vi "MTIF_Read_Smart.vi"(8 "error in":errorcluster, 9 "Input Parameters":T3={"Drop Bits"=0, "Output Files?"=TRUE, "STD Threshold Ratio for Start"=1.2, "STD Threshold Ratio for Stop"=1.1, "Output Image Type"=0, "Timeout for Queue(ms)"=1000, "Output Queue?"=FALSE, "Output File Format"=enum."TIFF", "Initial STD Threshold"=65535.0, "Number of Buffered Frames"=150, "Centroid Distence Threshold"=1.0} {"Output Image Type" items=["Grayscale (U8)", "Grayscale (I16)", "Grayscale (SGL)", "Complex (CSG)", "RGB (U32)", "HSL (U32)", "RGB (U64)", "Grayscale (U16)"]}, 10 "File Name (.mtif)":string="zebrafish_7", 11 "Folder Path":path=path "X:/Zebrafish_VR_Data") -> (0 "error out":errorcluster, 2 "Manual ROI":T1={"Global Rectangle"=[143, 107, 365, 263], "Contours"=[{"Contour Type"=0, "ROI Type"=4, "Points"=[143, 107, 365, 263]}]}, 3 "U16 Array Queue Out":refnum<queue>)   [LabVIEW 2014]
uses:
  <vilib>/vision/NI_Vision_Development_Module.lvlib
panel:
  out "Buffer Full?":bool=TRUE
  out "Standard Variation":sgl=42.84885
  out "Centroid":cluster{"X Centroid":sgl, "Y Centroid":sgl}={"X Centroid"=249.5989, "Y Centroid"=187.47522} {"Y Centroid" format="%.2f"; "X Centroid" format="%.2f"}
  in  "Stop":bool
  out "Frame No.":i32=996
  out "Sequence No.":u16
  out "Progress":dbl=1.0000000032682703 format="%#.3f"
  out "Data Valid?":bool=TRUE
  out "Raw Image":T4(plugin-control)
  out "Frame Rate":dbl=550.0
  out "File ROI":T5={"Left"=0, "Top"=0, "Right"=639, "Bottom"=479, "Rotation"=0.0} {"Rotation" format="%.2f"; "Left" scale=0.0..1024.0; "Right" scale=0.0..1024.0}
  # "Max 2GB\nfor one AVI file!"
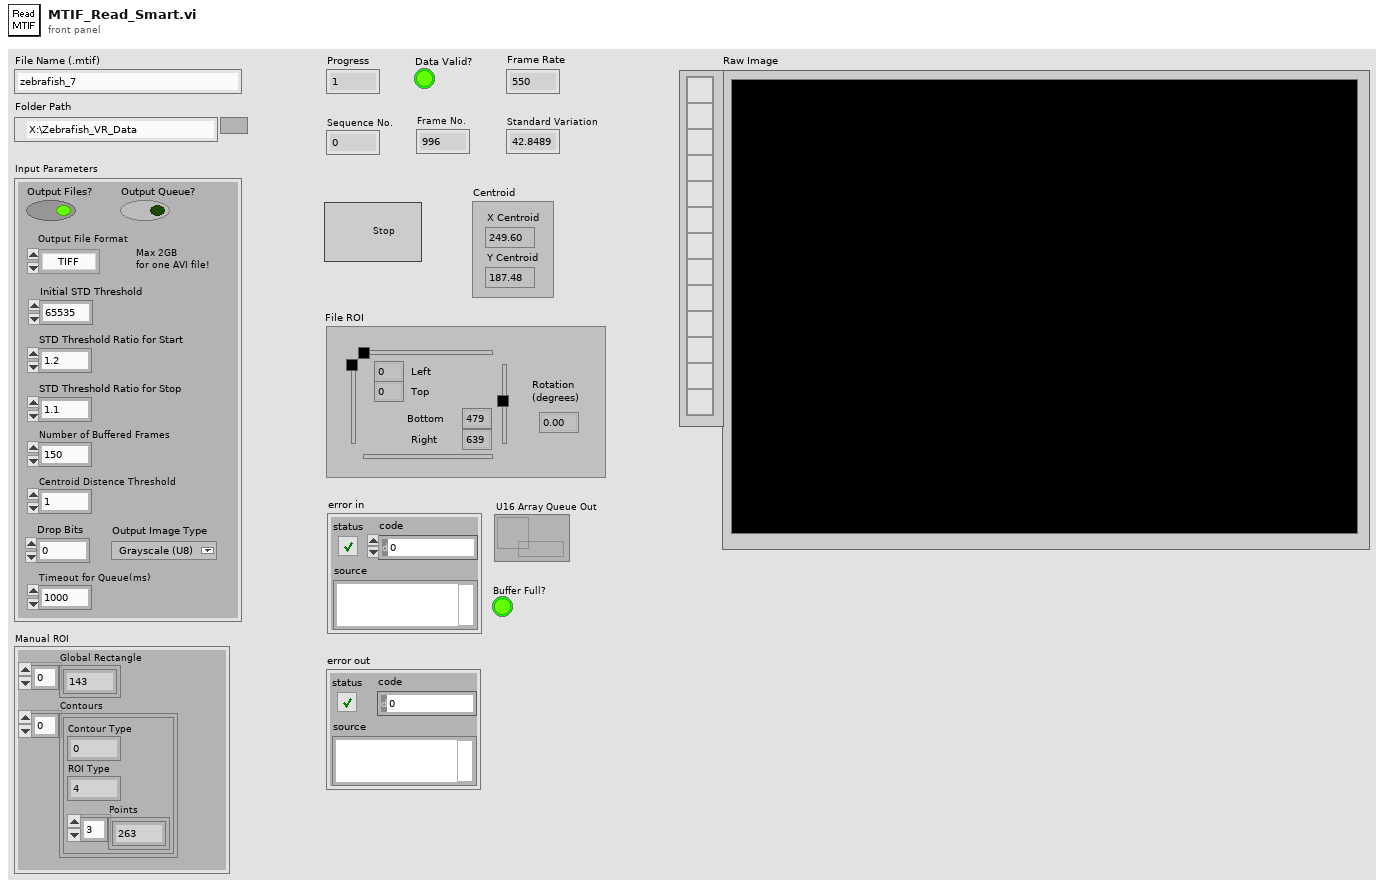
[diagram p1: front panel]
types:
  T1 = cluster{"Global Rectangle":i32[], "Contours":cluster{"Contour Type":u32, "ROI Type":u32, "Points":i32[]}[]}
  T2 = typedef "Image Type" = u32
  T3 = cluster{"Drop Bits":i8, "Output Files?":bool, "STD Threshold Ratio for Start":dbl, "STD Threshold Ratio for Stop":dbl, "Output Image Type":T2, "Timeout for Queue(ms)":u32, "Output Queue?":bool, "Output File Format":enum16{"TIFF", "AVI"}, "Initial STD Threshold":sgl, "Number of Buffered Frames":i32, "Centroid Distence Threshold":sgl}
  T4 = typedef "IMAQ Image.ctl" = refnum<image>
  T5 = typedef "IMAQ Rectangle" = cluster{"Left":i32, "Top":i32, "Right":i32, "Bottom":i32, "Rotation":dbl}
  T6 = cluster{"ImgDataArray":u16[][], "Centroid":cluster{"X Centroid":sgl, "Y Centroid":sgl}, "Frame No.":i32, "Standard Variation":sgl}
  T7 = enum16{"big-endian, network order", "native, host order", "little-endian"}
  T8 = enum16{"open", "replace", "create", "open or create", "replace or create", "replace or create with confirmation"}
  T9 = cluster{"[0]":i32, "[1]":i32, "[2]":i32, "[3]":i32}
  T10 = cluster{"Global Rectangle":i32[], "Contours":cluster{"Contour Type":u32, "Type":u32, "Coordinates":i32[]}[]}
  T11 = cluster{"Mean Value":sgl, "Standard Variation":sgl, "Minimal Value":sgl, "Maximal Value":sgl, "Area (calibrated)":sgl, "Area (pixels)":u32, "%":sgl, "Calibration Valid":bool}
  T12 = typedef "IMAQ AVI2 Refnum.ctl" = refnum<k20>
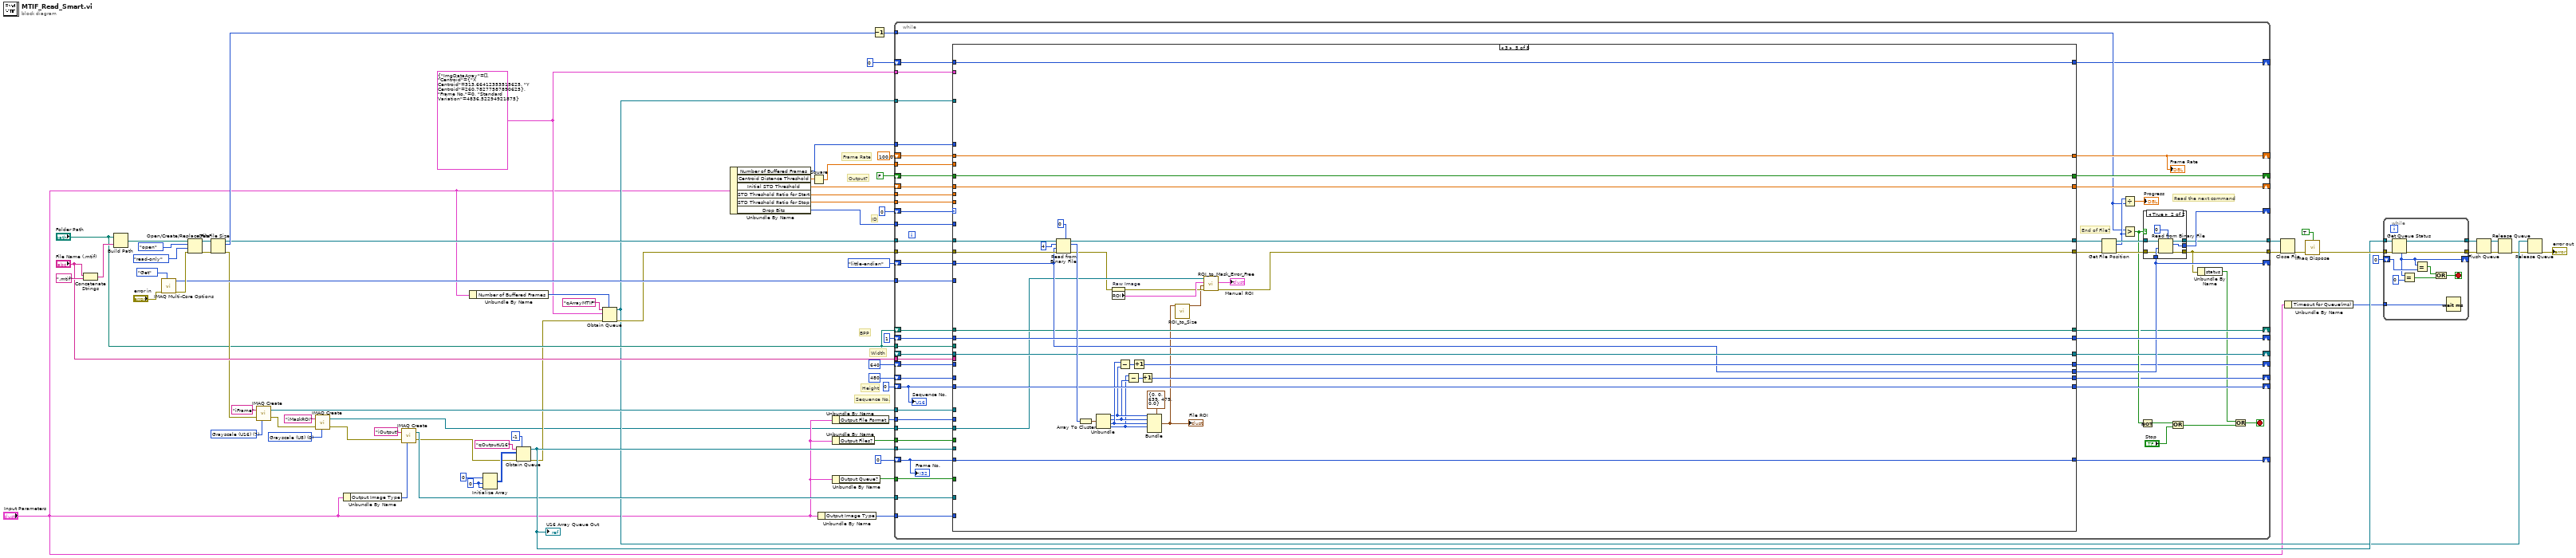
[diagram p0: block diagram]
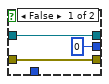
[diagram p2: hidden frame]
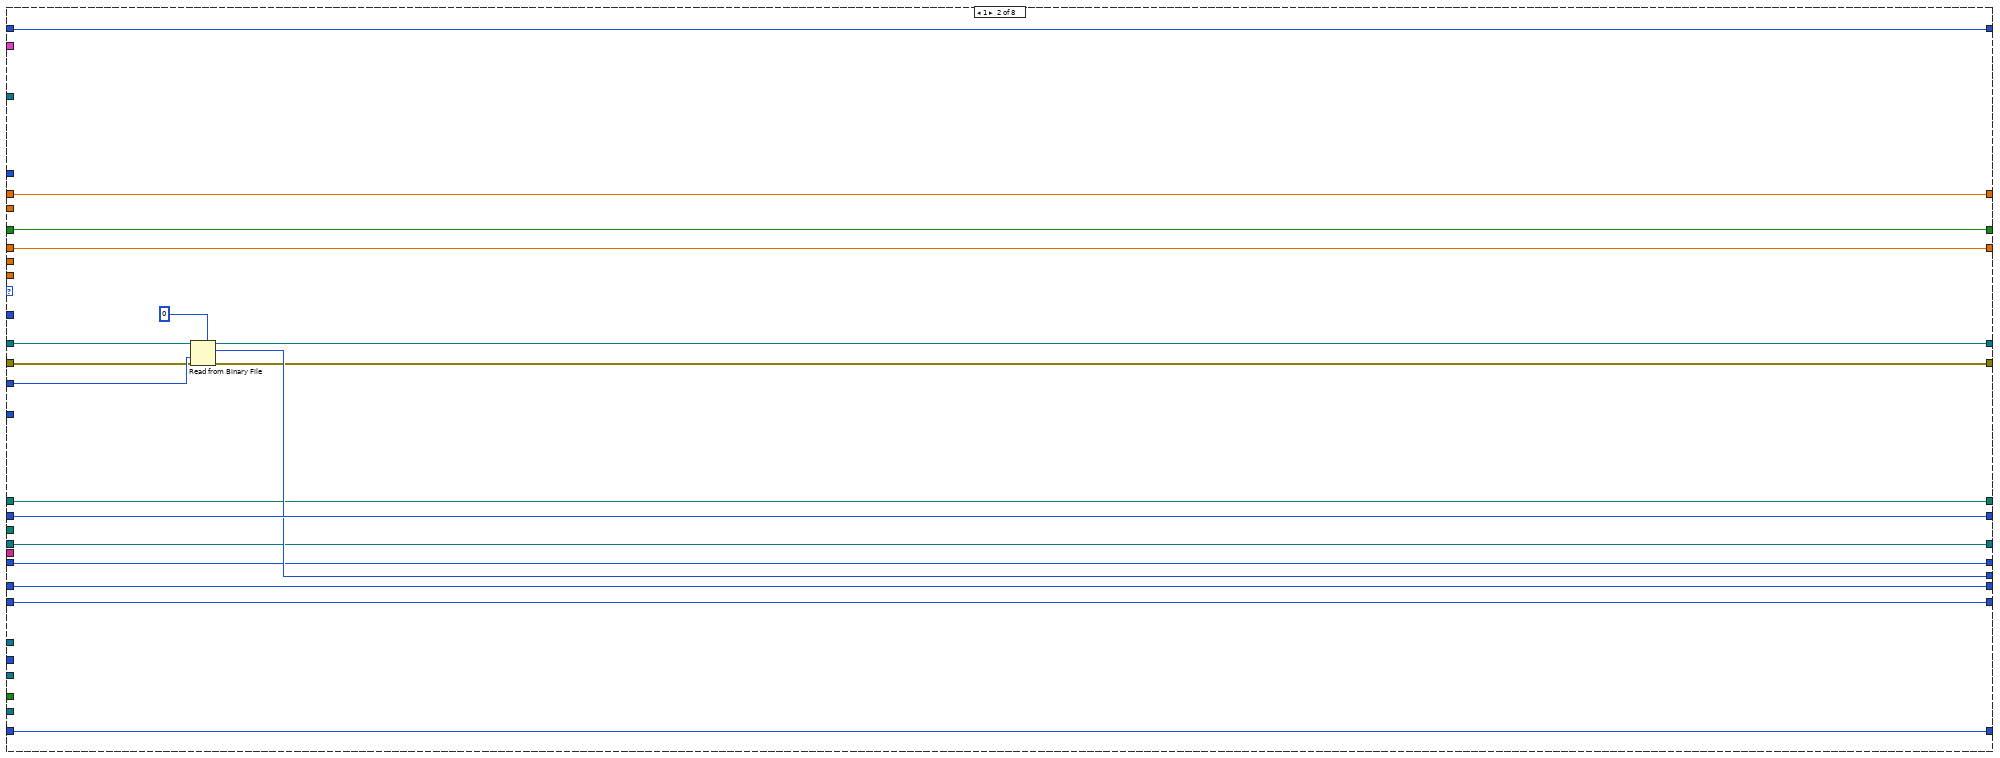
[diagram p4: hidden frame]
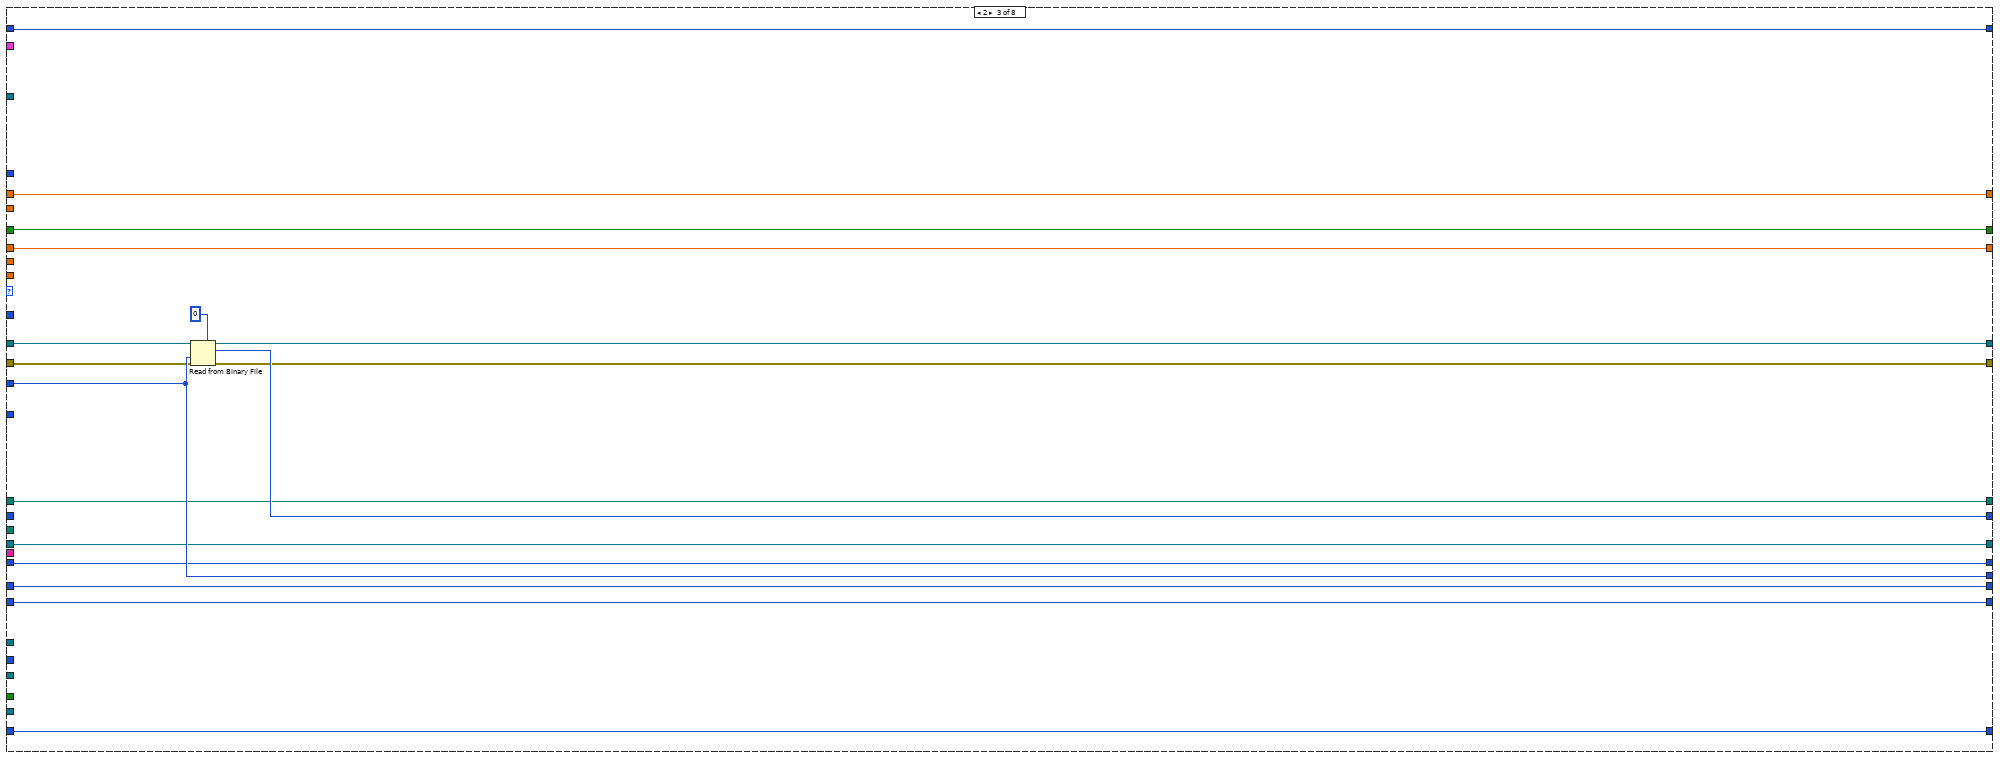
[diagram p5: hidden frame]
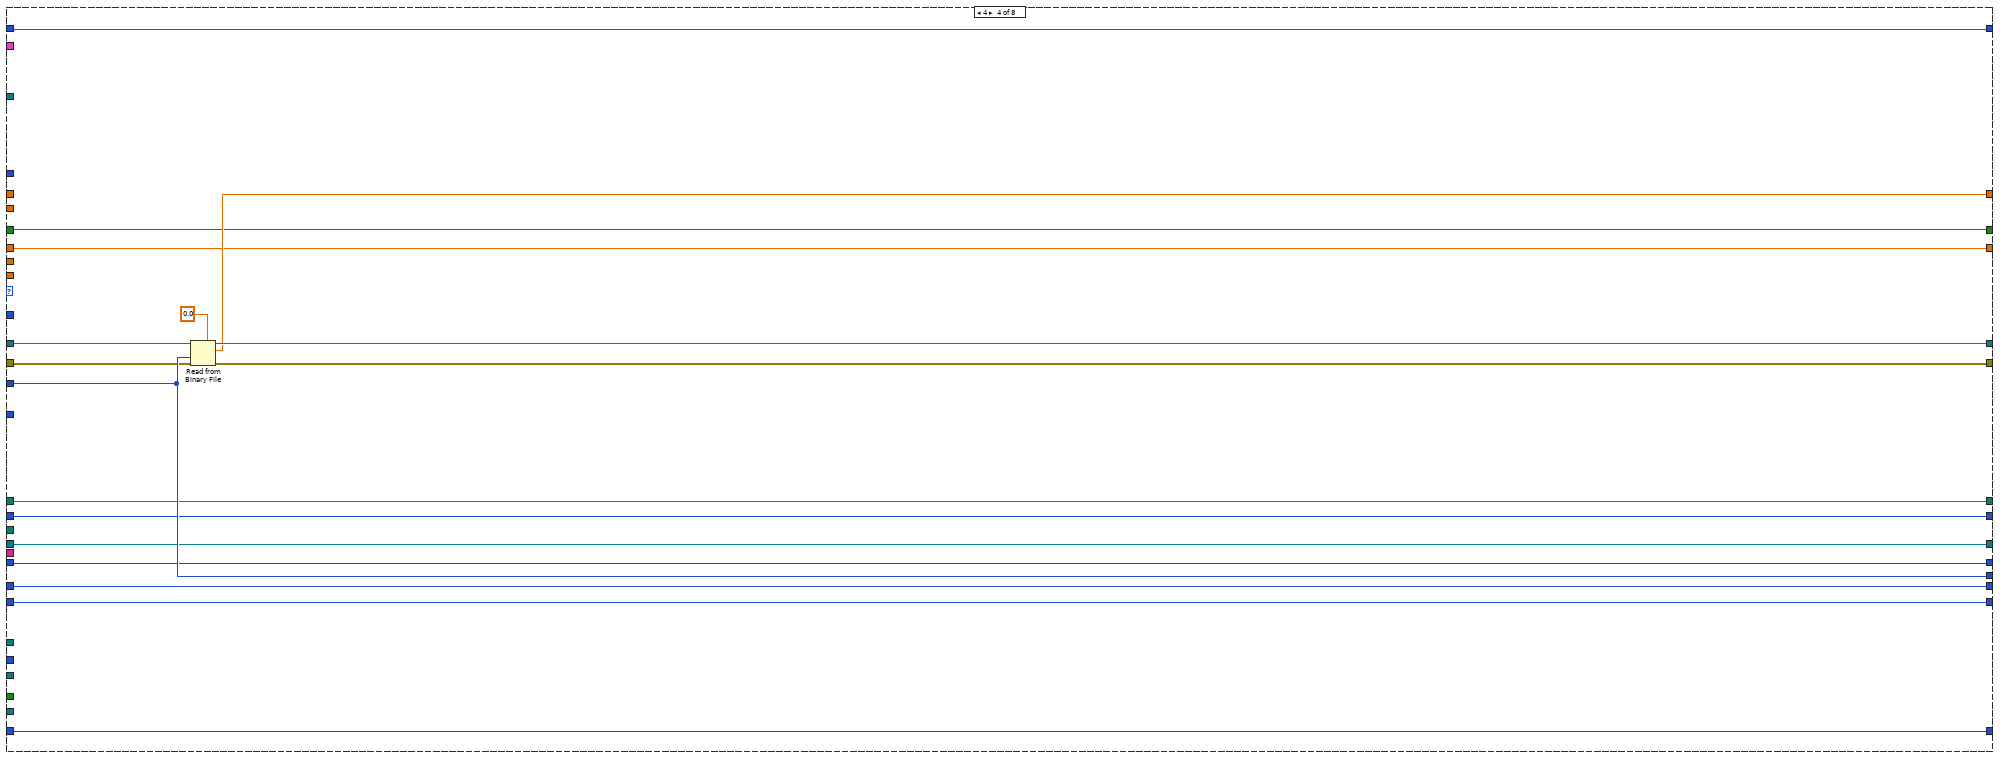
[diagram p6: hidden frame]
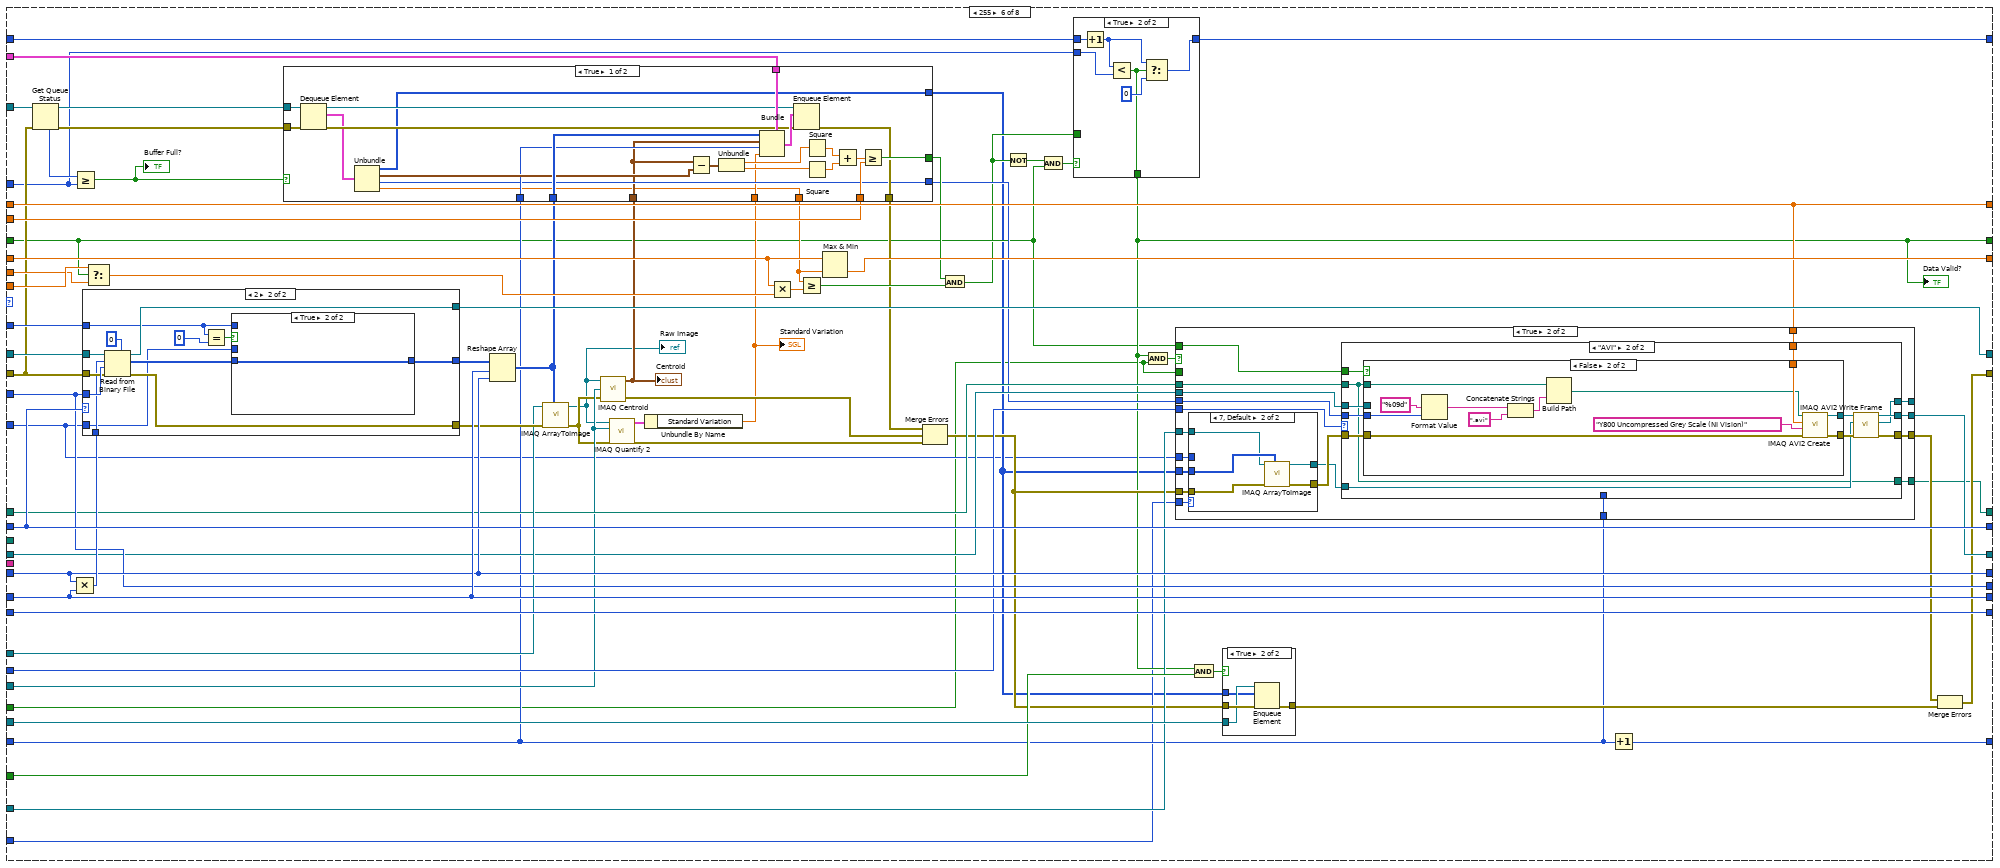
[diagram p7: hidden frame]
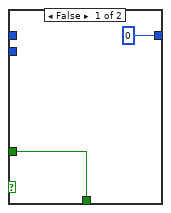
[diagram p8: hidden frame]
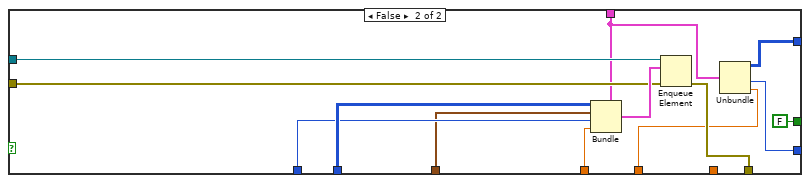
[diagram p9: hidden frame]
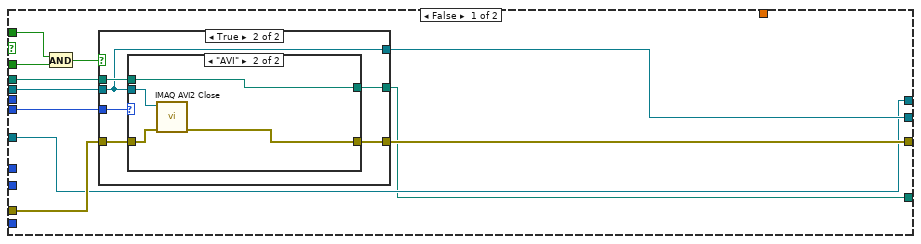
[diagram p11: hidden frame]
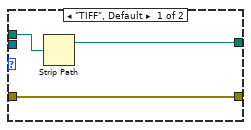
[diagram p13: hidden frame]
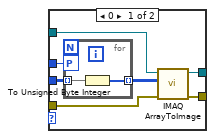
[diagram p14: hidden frame]
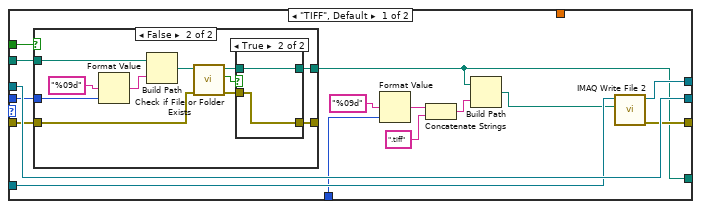
[diagram p15: hidden frame]
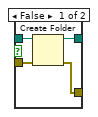
[diagram p17: hidden frame]
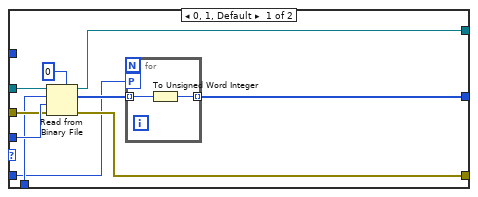
[diagram p19: hidden frame]
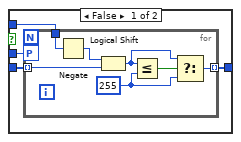
[diagram p20: hidden frame]
diagram:
  w13 = T6 {"ImgDataArray"=[], "Centroid"={"X Centroid"=313.66412, "Y Centroid"=260.78278}, "Frame No."=0, "Standard Variation"=4836.523}
  w24 = T2 0 items=["Grayscale (U8)", "Grayscale (I16)", "Grayscale (SGL)", "Complex (CSG)", "RGB (U32)", "HSL (U32)", "RGB (U64)", "Grayscale (U16)"] ("Image Type")
  w25 = T2 7 items=["Grayscale (U8)", "Grayscale (I16)", "Grayscale (SGL)", "Complex (CSG)", "RGB (U32)", "HSL (U32)", "RGB (U64)", "Grayscale (U16)"] ("Image Type")
  w20 = 0 ("dimension size")
  # "Output?"
  # "Sequence No."
  # "Height"
  # "Width"
  # "BPP"
  # "ID"
  # "Frame Rate"
  n1 = Concatenate Strings("File Name (.mtif)", ".mtif" ("string")) -> (w73:string)
  n2 = Build Path(base path="Folder Path", name or relative path=w73) -> (appended path=w69:path)
  n3 = call "IMAQ Multi-Core Options"("Get/Set Number of Cores (Get)"=enum32{"Get", "Set", "Set Max Available"}."Get", "error in (no error)"="error in") -> ("error out"=w59:errorcluster, "Cores Utilized"=w58:u32)  [unwired: 8 in]
  n4 = Open/Create/Replace File(file path (use dialog)=w69, error in=w59, operation (0:open)=T8."open", access (0:read/write)=enum16{"read/write", "read-only", "write-only"}."read-only") -> (refnum out=w64:refnum<file>, error out=w65:errorcluster)  [unwired: 2 in, 1 out]
  n5 = Get File Size(file=w64, error in=w65) -> (refnum out=w55:refnum<file>, size (in bytes)=w63:i64, 0:w53:errorcluster)
  n6 = call "IMAQ Create"("Image Name"="iFrame", "Image Type"=w25, "error in (no error)"=w53) -> ("New Image"=w52:T4, "error out"=w51:errorcluster)  [unwired: 2 in]
  n7 = call "IMAQ Create"("Image Name"="iMaskROI", "Image Type"=w24, "error in (no error)"=w51) -> ("New Image"=w2:T4, "error out"=w3:errorcluster)  [unwired: 2 in]
  n8 = Unbundle By Name("Input Parameters") -> ("Output Image Type"=w22:T2)
  n9 = call "IMAQ Create"("Image Name"="iOutput", "Image Type"=w22, "error in (no error)"=w3) -> ("New Image"=w21:T4, "error out"=w1:errorcluster)  [unwired: 2 in]
  n10 = Unbundle By Name("Input Parameters") -> ("Number of Buffered Frames"=w15:i32)
  n11 = Initialize Array(u16 0 ("element"), w20, w20) -> (w44:u16[][])
  n12 = Obtain Queue(max queue size (-1, unlimited)=-1, name (unnamed)="qOutputU16", element data type=w44, error in (no error)=w1) -> (queue out=w35:refnum<queue>, error out=w16:errorcluster)  [unwired: 1 in, 1 out]
  "U16 Array Queue Out" <- w35
  n13 = Obtain Queue(max queue size (-1, unlimited)=w15, name (unnamed)="qArrayMTIF", element data type=w13, error in (no error)=w16) -> (queue out=w9:refnum<queue>, error out=w14:errorcluster)  [unwired: 1 in, 1 out]
  n14 = Unbundle By Name("Input Parameters") -> ("Number of Buffered Frames"=w18:i32, "Centroid Distence Threshold"=w11:sgl, "Initial STD Threshold"=w19:sgl, "STD Threshold Ratio for Start"=w32:dbl, "STD Threshold Ratio for Stop"=w30:dbl, "Drop Bits"=w29:i8)
  n15 = Square(x=w11) -> (x^2=w10:sgl)
  n16 = Unbundle By Name("Input Parameters") -> ("Output Image Type"=w4:T2)
  n17 = Unbundle By Name("Input Parameters") -> ("Output File Format"=w28:enum16{"TIFF", "AVI"})
  n18 = Unbundle By Name("Input Parameters") -> ("Output Files?"=w34:bool)
  n19 = Unbundle By Name("Input Parameters") -> ("Output Queue?"=w33:bool)
  n20 = Decrement(x=w63) -> (x-1=w62:i64)
  n21 = while {
    shift-right: [w130] -> _
    shift-left: u8 0 -> [w137]
    shift-right: [w135] -> _
    shift-left: u8 1 -> [w136]
    tunnel: w55 -> [w134]
    shift-right: [w132] -> _
    shift-left: T7."little-endian" ("Byte Order") -> [w133]
    tunnel: w14 -> [w131]
    tunnel: [w80] -> w47
    shift-right: [w128] -> _
    shift-left: 100.0 -> [w129]
    shift-right: [w122] -> _
    shift-left: u16 0 -> [w127]
    shift-right: [w124] -> _
    shift-left: _ -> [w123]
    tunnel: w62 -> [w100]
    shift-right: [w116] -> _
    shift-left: 640 -> [w114]
    shift-right: [w115] -> _
    shift-left: 480 -> [w113]
    tunnel: w29 -> [w112]
    tunnel: w58 -> [w111]
    tunnel: w52 -> [w110]
    tunnel: w34 -> [w102]
    tunnel: w2 -> [w109]
    shift-right: [w106] -> _
    shift-left: w19 -> [w107]
    shift-right: [w104] -> _
    shift-left: FALSE -> [w108]
    tunnel: w30 -> [w105]
    tunnel: w32 -> [w103]
    tunnel: [w98] -> w46
    tunnel: "Folder Path" -> [w126]
    tunnel: w35 -> [w97]
    tunnel: w33 -> [w96]
    tunnel: w28 -> [w95]
    tunnel: "File Name (.mtif)" -> [w125]
    shift-right: [w93] -> _
    shift-left: "Folder Path" -> [w94]
    tunnel: w21 -> [w90]
    tunnel: w18 -> [w89]
    tunnel: w10 -> [w88]
    tunnel: w9 -> [w87]
    tunnel: w13 -> [w86]
    shift-right: [w84] -> _
    shift-left: 0 -> [w85]
    shift-right: [w82] -> _
    shift-left: 0 -> [w83]
    tunnel: w4 -> [w81]
    stop <- w77 stop-if-true
    # "Read the next command"
    # "End of File?"
    n22 = case shown="3" w137 {
      tunnel: w133 -> [w161 w178 w195 w212 w224 w305 w535 w597]
      tunnel: [w161 w174 w195 w212 w224 w305 w535 w597] -> w132
      tunnel: w136 -> [w160 w177 _ w206 w238 w314 w553 w592]
      tunnel: [w160 w177 w192 w206 w238 w314 w553 w592] -> w135
      tunnel: w134 -> [w159 w176 w193 w210 w245 w316 w543 w595]
      tunnel: w131 -> [w158 w175 w194 w211 w246 w272 w526 w586]
      tunnel: [w158 w173 w191 w209 w221 w290 w547 w601] -> w120
      tunnel: [w159 w172 w190 w208 w244 w304 w542 w594] -> w121
      tunnel: [w157 w171 w189 w207 w239 w293 w548 w577] -> w128
      tunnel: w129 -> [w157 w171 w189 _ w239 w293 w548 w577]
      tunnel: w127 -> [w155 w169 w187 w204 w236 w315 w532 w590]
      tunnel: w126 -> [_ _ _ _ _ _ w551 _]
      tunnel: w125 -> [_ _ _ _ _ _ w550 _]
      tunnel: [w156 w170 w188 w205 w237 w299 w531 w578] -> w124
      tunnel: w123 -> [w156 w170 w188 w205 w237 w300 w531 w578]
      tunnel: [w155 w169 w187 w204 w236 w315 w532 w589] -> w122
      tunnel: [w154 w168 w186 w203 w229 w309 w545 w599] -> w116
      tunnel: [w153 w167 w185 w202 w228 w310 w546 w600] -> w115
      tunnel: w114 -> [w154 w168 w186 w203 _ w309 w545 w599]
      tunnel: w113 -> [w153 w167 w185 w202 _ w310 w546 w600]
      tunnel: w112 -> [_ _ _ _ _ w313 _ _]
      tunnel: w111 -> [_ _ _ _ _ w249 _ w569]
      tunnel: w110 -> [_ _ _ _ _ w307 _ _]
      tunnel: w109 -> [_ _ _ _ w220 w283 _ _]
      tunnel: w108 -> [w152 w166 w184 w201 w227 w253 _ w582]
      tunnel: w107 -> [w151 w165 w183 w200 w226 w296 w528 w593]
      tunnel: [w151 w165 w183 w200 w226 w303 w528 w593] -> w106
      tunnel: w105 -> [_ _ _ _ _ w302 _ _]
      tunnel: [w152 w166 w184 w201 w227 w254 FALSE FALSE] -> w104
      tunnel: w103 -> [_ _ _ _ _ w301 _ _]
      tunnel: w102 -> [_ _ _ _ _ w248 w534 w576]
      tunnel: w85 -> [w150 w164 w182 w199 w225 w265 _ w591]
      tunnel: [w150 w164 w182 w199 w225 w294 0 w591] -> w84
      tunnel: w97 -> [_ _ _ _ _ w292 _ w574]
      tunnel: w96 -> [_ _ _ _ _ w287 _ w575]
      tunnel: w95 -> [_ _ _ _ _ w286 _ w579]
      tunnel: w94 -> [w149 w163 w181 w198 w223 w285 _ w570]
      tunnel: [w149 w163 w181 w198 w223 w284 w529 w570] -> w93
      tunnel: w90 -> [_ _ _ _ _ w267 _ w573]
      tunnel: w89 -> [_ _ _ _ _ w255 _ _]
      tunnel: w88 -> [_ _ _ _ _ w277 _ _]
      tunnel: w87 -> [_ _ _ _ _ w274 w527 w587]
      tunnel: w86 -> [_ _ _ _ _ w263 _ _]
      tunnel: w83 -> [w148 w162 w180 w197 w222 w257 _ _]
      tunnel: [w148 w162 w180 w197 w222 w256 0 ("f") 0 ("f")] -> w82
      tunnel: w81 -> [_ _ _ _ _ w251 _ w580]
      frame 0, Default {
      }
      frame 1 {
        n23 = Read from Binary File(5:u8 0, 8:w175, 9:w178, 11:w176) -> (0:w173:errorcluster, 2:w174:u8, 3:w172:refnum<file>)  [unwired: 2 in, 1 out]
      }
      frame 2 {
        n24 = Read from Binary File(5:u8 0, 8:w194, 9:w195, 11:w193) -> (0:w191:errorcluster, 2:w192:u8, 3:w190:refnum<file>)  [unwired: 2 in, 1 out]
      }
      frame 4 {
        n25 = Read from Binary File(5:0.0, 8:w211, 9:w212, 11:w210) -> (0:w209:errorcluster, 2:w207:dbl, 3:w208:refnum<file>)  [unwired: 2 in, 1 out]
      }
      frame 3 {
        n26 = Read from Binary File(5:0, 8:w246, 9:w224, 10:4 ("count (1)"), 11:w245) -> (0:w217:errorcluster, 2:w242:i32[], 3:w244:refnum<file>)  [unwired: 1 in, 1 out]
        n27 = Array To Cluster(array=w242) -> (cluster=w241:T9)
        n28 = Unbundle(w241) -> ("[0]"=w232:i32, "[1]"=w231:i32, "[2]"=w233:i32, "[3]"=w230:i32)
        n29 = property on="Raw Image" class="ImageControl"(error in=w217) -> (error out=w216:errorcluster, "ROI"=w219:T1)  [unwired: 1 in, 1 out]
        n30 = Subtract(x=w233, y=w232) -> (x-y=w234:i32)
        n31 = Subtract(x=w230, y=w231) -> (x-y=w235:i32)
        n32 = Increment(x=w234) -> (x+1=w229:i32)
        n33 = Increment(x=w235) -> (x+1=w228:i32)
        n34 = Bundle(cluster=T5 {"Left"=0, "Top"=0, "Right"=639, "Bottom"=479, "Rotation"=0.0} ("Actual ROI"), "Left"=w232, "Top"=w231, "Right"=w233, "Bottom"=w230) -> (w215:T5)  [unwired: 1 in]
        "File ROI" <- w215
        n35 = call "ROI_to_Size.vi"("Actual ROI"=w215) -> ("Image Size"=w214:cluster{"X":i32, "Y":i32})  [unwired: 10 in]
        n36 = call "ROI_to_Mask_Error_Free.vi"("error in (no error)"=w216, "Image Size"=w214, "ROI in"=w219, "Refnum in"=w220) -> ("error out"=w221:errorcluster, "ROI out"=→"Manual ROI":T10)  [unwired: 5 in, 1 out]
      }
      frame 255 {
        n37 = Get Queue Status(queue=w274, error in (no error)=w272) -> (queue out=w271:refnum<queue>, error out=w270:errorcluster, # elements in queue=w273:i32)  [unwired: 1 in, 5 out]
        n38 = Multiply(x=w309, y=w310) -> (x*y=w312:i32)
        n39 = Greater Or Equal?(x=w273, y=w255) -> (x >= y?=w262:bool)
        "Buffer Full?" <- w262
        n40 = case shown="2" w314 {
          tunnel: w305 -> [w494 w509]
          tunnel: w272 -> [w493 w508]
          tunnel: w316 -> [w492 w507]
          tunnel: [w491 w505] -> w308
          tunnel: [w490 w503] -> w304
          tunnel: [w487 w501] -> w311
          tunnel: w313 -> [_ w499]
          tunnel: w312 -> [w489 w504]
          tunnel: w249 -> [w486 w502]
          frame 0, 1, Default {
            n41 = Read from Binary File(5:u8 0, 8:w493, 9:w494, 10:w489, 11:w492) -> (0:w491:errorcluster, 2:w488:u8[], 3:w490:refnum<file>)  [unwired: 1 in, 1 out]
            n42 = for {
              workers-P: w486 -> [_]
              tunnel: [w497] -> w487 mode=indexing
              tunnel: w488 -> [w496] mode=indexing
              n43 = To Unsigned Word Integer(number=w496) -> (unsigned 16bit integer=w497:u16)
            }
          }
          frame 2 {
            n44 = Read from Binary File(5:u16 0, 8:w508, 9:w509, 10:w504, 11:w507) -> (0:w505:errorcluster, 2:w506:u16[], 3:w503:refnum<file>)  [unwired: 1 in, 1 out]
            n45 = Equal?(x=w499, y=i8 0) -> (x = y?=w500:bool)
            n46 = case shown="True" w500 {
              tunnel: w506 -> [w514 w522]
              tunnel: w499 -> [w513 _]
              tunnel: w502 -> [w512 _]
              tunnel: [w511 w522] -> w501
              frame False {
                n47 = for {
                  tunnel: w514 -> [w516] mode=indexing
                  tunnel: w513 -> [w518]
                  workers-P: w512 -> [_]
                  tunnel: [w515] -> w511 mode=indexing
                  w520 = u16 255 ("y")
                  n48 = Negate(x=w518) -> (-x=w517:i8)
                  n49 = Logical Shift(y=w517, x=w516) -> (x << y=w519:u16)
                  n50 = Less Or Equal?(x=w519, y=w520) -> (x <= y?=w521:bool)
                  n51 = Select(t=w519, s=w521, f=w520) -> (s? t:f=w515:u16)
                }
              }
              frame True {
              }
            }
          }
        }
        n52 = Select(t=w302, s=w253, f=w301) -> (s? t:f=w295:dbl)
        n53 = Reshape Array(w311, w310, w309) -> (w275:u16[][])
        n54 = call "IMAQ ArrayToImage"("Image Pixels (U16)"=w275, "error in (no error)"=w308, "Image"=w307) -> ("error out"=w282:errorcluster, "Image Out"=w268:T4)  [unwired: 7 in]
        "Raw Image" <- w268
        n55 = call "IMAQ Centroid"("error in (no error)"=w282, "Image Mask"=w283, "Image"=w268) -> ("error out"=w280:errorcluster, "Centroid"=w276:cluster{"X Centroid":sgl, "Y Centroid":sgl})  [unwired: 1 in]
        "Centroid" <- w276
        n56 = call "IMAQ Quantify 2"("error in (no error)"=w282, "Image Mask"=w283, "Image"=w268) -> ("error out"=w281:errorcluster, "Global Report"=w306:T11)  [unwired: 6 in, 1 out]
        n57 = Unbundle By Name(w306) -> ("Standard Variation"=w261:sgl)
        "Standard Variation" <- w261
        n58 = case shown="True" w262 {
          tunnel: [w342 FALSE] -> w278
          tunnel: w277 -> [w341 _]
          tunnel: w276 -> [w327 w357]
          tunnel: w275 -> [w340 w361]
          tunnel: w271 -> [w338 w356]
          tunnel: w270 -> [w337 w355]
          tunnel: w263 -> [w336 w354]
          tunnel: [w333 w359] -> w269
          tunnel: [w331 w353] -> w250
          tunnel: w265 -> [w330 w358]
          tunnel: [w329 w351] -> w264
          tunnel: w261 -> [w326 w350]
          tunnel: [w325 w349] -> w260
          frame True {
            n59 = Dequeue Element(queue=w338, error in (no error)=w337) -> (queue out=w334:refnum<queue>, element=w328:T6, error out=w335:errorcluster)  [unwired: 1 in, 1 out]
            n60 = Unbundle(w328) -> ("ImgDataArray"=w331:u16[][], "Centroid"=w332:cluster{"X Centroid":sgl, "Y Centroid":sgl}, "Frame No."=w329:i32, "Standard Variation"=w325:sgl)
            n61 = Subtract(x=w327, y=w332) -> (x-y=w348:cluster{"X Centroid":sgl, "Y Centroid":sgl})
            n62 = Unbundle(w348) -> ("X Centroid"=w347:sgl, "Y Centroid"=w346:sgl)
            n63 = Bundle(cluster=w336, "ImgDataArray"=w340, "Centroid"=w327, "Frame No."=w330, "Standard Variation"=w326) -> (w339:T6)
            n64 = Enqueue Element(queue=w334, element=w339, error in (no error)=w335) -> (error out=w333:errorcluster)  [unwired: 1 in, 2 out]
            n65 = Square(x=w347) -> (x^2=w345:sgl)
            n66 = Square(x=w346) -> (x^2=w344:sgl)
            n67 = Add(x=w345, y=w344) -> (x+y=w343:sgl)
            n68 = Greater Or Equal?(x=w343, y=w341) -> (x >= y?=w342:bool)
          }
          frame False {
            n69 = Bundle(cluster=w354, "ImgDataArray"=w361, "Centroid"=w357, "Frame No."=w358, "Standard Variation"=w350) -> (w360:T6)
            n70 = Enqueue Element(queue=w356, element=w360, error in (no error)=w355) -> (error out=w359:errorcluster)  [unwired: 1 in, 2 out]
            n71 = Unbundle(w354) -> ("ImgDataArray"=w353:u16[][], "Frame No."=w351:i32, "Standard Variation"=w349:sgl)  [unwired: 1 out]
          }
        }
        n72 = Multiply(x=w296, y=w295) -> (x*y=w297:dbl)
        n73 = Greater Or Equal?(x=w260, y=w297) -> (x >= y?=w279:bool)
        n74 = Max & Min(x=w296, y=w260) -> (min(x,y)=w303:sgl)  [unwired: 1 out]
        n75 = Merge Errors(w269, w280, w281) -> (w266:errorcluster)
        n76 = And(x=w278, y=w279) -> (x .and. y?=w252:bool)
        n77 = Not(x=w252) -> (.not. x?=w259:bool)
        n78 = And(x=w259, y=w253) -> (x .and. y?=w258:bool)
        n79 = case shown="True" w258 {
          tunnel: w257 -> [_ w324]
          tunnel: [0 w322] -> w256
          tunnel: w255 -> [_ w320]
          tunnel: [w317 w319] -> w254
          tunnel: w252 -> [w317 _]
          frame False {
          }
          frame True {
            n80 = Increment(x=w324) -> (x+1=w321:i32)
            n81 = Less?(x=w321, y=w320) -> (x < y?=w319:bool)
            n82 = Select(t=w321, s=w319, f=0) -> (s? t:f=w322:i32)
          }
        }
        "Data Valid?" <- w254
        n83 = And(x=w254, y=w248) -> (x .and. y?=w298:bool)
        n84 = case shown="True" w298 {
          tunnel: w266 -> [w376 w400]
          tunnel: w267 -> [w372 w398]
          tunnel: [w375 w411] -> w289
          tunnel: w300 -> [w377 w407]
          tunnel: [w374 w410] -> w299
          tunnel: w293 -> [_ w409]
          tunnel: w285 -> [w371 w408]
          tunnel: w264 -> [_ w406]
          tunnel: w286 -> [w373 w405]
          tunnel: [w372 w404] -> _
          tunnel: [w370 w403] -> w284
          tunnel: w265 -> [_ w402]
          tunnel: w250 -> [_ w401]
          tunnel: w253 -> [w369 w396]
          tunnel: w251 -> [_ w395]
          tunnel: w249 -> [_ w394]
          tunnel: w248 -> [w367 _]
          frame False {
            n85 = And(x=w369, y=w367) -> (x .and. y?=w368:bool)
            n86 = case shown="True" w368 {
              tunnel: w377 -> [w379 w382]
              tunnel: w376 -> [w380 w385]
              tunnel: [w380 w384] -> w375
              tunnel: [w379 w382] -> w374
              tunnel: w373 -> [_ w386]
              tunnel: w371 -> [w378 w383]
              tunnel: [w378 w381] -> w370
              frame False {
              }
              frame True {
                n87 = case shown="\"AVI\"" w386 {
                  tunnel: w382 -> [_ w393]
                  tunnel: w385 -> [w387 w392]
                  tunnel: [w387 w391] -> w384
                  tunnel: w383 -> [w389 w390]
                  tunnel: [w388 w390] -> w381
                  frame "TIFF", Default {
                    n88 = Strip Path(path=w389) -> (stripped path=w388:path)  [unwired: 1 out]
                  }
                  frame "AVI" {
                    n89 = call "IMAQ AVI2 Close"("error in (no error)"=w392, "AVI Refnum"=w393) -> ("error out"=w391:errorcluster)  [unwired: 9 in]
                  }
                }
              }
            }
          }
          frame True {
            n90 = case shown="7, Default" w395 {
              tunnel: w401 -> [w414 w425]
              tunnel: w400 -> [w418 w424]
              tunnel: [w417 w423] -> w399
              tunnel: w398 -> [w416 w422]
              tunnel: [w415 w421] -> w397
              tunnel: w394 -> [w412 _]
              frame 0 {
                n91 = for {
                  workers-P: w412 -> [_]
                  tunnel: [w420] -> w413 mode=indexing
                  tunnel: w414 -> [w419] mode=indexing
                  n92 = To Unsigned Byte Integer(number=w419) -> (unsigned 8bit integer=w420:u8[])
                }
                n93 = call "IMAQ ArrayToImage"("error in (no error)"=w418, "Image Pixels (U8)"=w413, "Image"=w416) -> ("error out"=w417:errorcluster, "Image Out"=w415:T4)  [unwired: 7 in]
              }
              frame 7, Default {
                n94 = call "IMAQ ArrayToImage"("Image Pixels (U16)"=w425, "error in (no error)"=w424, "Image"=w422) -> ("error out"=w423:errorcluster, "Image Out"=w421:T4)  [unwired: 7 in]
              }
            }
            n95 = case shown="\"AVI\"" w405 {
              tunnel: [w436 w471] -> w411
              tunnel: [w440 w470] -> w410
              tunnel: w399 -> [w437 w469]
              tunnel: w409 -> [_ w468]
              tunnel: w396 -> [w439 w466]
              tunnel: w408 -> [w435 w460]
              tunnel: w406 -> [w438 w464]
              tunnel: w407 -> [w440 w463]
              tunnel: w397 -> [w434 w462]
              tunnel: [w433 w461] -> w404
              tunnel: [w430 w460] -> w403
              tunnel: w402 -> [w431 _]
              frame "TIFF", Default {
                n96 = case shown="False" w439 {
                  tunnel: w437 -> [w442 w449]
                  tunnel: [w442 w445] -> _
                  tunnel: w435 -> [w441 w453]
                  tunnel: w438 -> [_ w452]
                  tunnel: [w441 w443] -> w430
                  frame True {
                  }
                  frame False {
                    n97 = Format Value(format string="%09d", value (0)=w452) -> (output string=w444:string)  [unwired: 1 in]
                    n98 = Build Path(base path=w453, name or relative path=w444) -> (appended path=w450:path)
                    n99 = call <vilib>:"Check if File or Folder Exists.vi"("error in (no error)"=w449, "path"=w450) -> ("error out"=w446:errorcluster, "file or folder exists?"=w448:bool, "dup path"=w447:path)  [unwired: 7 in]
                    n100 = case shown="True" w448 {
                      tunnel: w447 -> [w457 w458]
                      tunnel: w446 -> [w456 w459]
                      tunnel: [w455 w459] -> w445
                      tunnel: [w454 w458] -> w443
                      frame False {
                        n101 = Create Folder(path (use dialog)=w457, error in=w456) -> (created path=w454:path, error out=w455:errorcluster)  [unwired: 1 in, 1 out]
                      }
                      frame True {
                      }
                    }
                  }
                }
                n102 = Format Value(format string="%09d", value (0)=w431) -> (output string=w428:string)  [unwired: 1 in]
                n103 = Concatenate Strings(w428, ".tiff" ("string")) -> (w427:string)
                n104 = Build Path(base path=w430, name or relative path=w427) -> (appended path=w426:path)
                n105 = call-poly "IMAQ Write File 2"("File Path"=w426, "Image"=w434) -> ("error out"=w436:errorcluster, "Image Out (duplicate)"=w433:T4)  [unwired: 8 in]
              }
              frame "AVI" {
                n106 = case shown="False" w466 {
                  tunnel: w469 -> [w473 w484]
                  tunnel: w468 -> [_ w483]
                  tunnel: [w473 w481] -> w467
                  tunnel: [w472 w482] -> w465
                  tunnel: w460 -> [_ w480]
                  tunnel: w464 -> [_ w476]
                  tunnel: w463 -> [w472 _]
                  frame True {
                  }
                  frame False {
                    n107 = Format Value(format string="%09d", value (0)=w476) -> (output string=w474:string)  [unwired: 1 in]
                    n108 = Concatenate Strings(w474, ".avi" ("string")) -> (w478:string)
                    n109 = Build Path(base path=w480, name or relative path=w478) -> (appended path=w479:path)
                    n110 = call "IMAQ AVI2 Create"("error in (no error)"=w484, "Codec"="Y800 Uncompressed Grey Scale (NI Vision)", "Frames Per Second"=w483, "AVI Path"=w479) -> ("error out"=w481:errorcluster, "AVI Refnum"=w482:T12)  [unwired: 6 in]
                  }
                }
                n111 = call "IMAQ AVI2 Write Frame"("error in (no error)"=w467, "Image"=w462, "AVI Refnum"=w465) -> ("error out"=w471:errorcluster, "Image Out (duplicate)"=w461:T4, "AVI Refnum (duplicate)"=w470:T12)  [unwired: 6 in]
              }
            }
          }
        }
        n112 = And(x=w254, y=w287) -> (x .and. y?=w288:bool)
        n113 = case shown="True" w288 {
          tunnel: w292 -> [_ w365]
          tunnel: w266 -> [w362 w366]
          tunnel: w250 -> [_ w364]
          tunnel: [w362 w363] -> w291
          frame False {
          }
          frame True {
            n114 = Enqueue Element(queue=w365, element=w364, error in (no error)=w366) -> (error out=w363:errorcluster)  [unwired: 1 in, 2 out]
          }
        }
        n115 = Increment(x=w265) -> (x+1=w294:i32)
        n116 = Merge Errors(w289, w291) -> (w290:errorcluster)
      }
      frame 6 {
        n117 = Flush Queue(queue=w527, error in (no error)=w526) -> (error out=w525:errorcluster)  [unwired: 2 out]
        n118 = Read from Binary File(5:0.0, 8:w525, 9:w535, 11:w543) -> (0:w541:errorcluster, 2:w540:dbl, 3:w542:refnum<file>)  [unwired: 2 in, 1 out]
        n119 = To Time Stamp(1:w540) -> (0:w538:timestamp)
        n120 = Format Date/Time String(time format string (%c)="%Y%m%d_%H%M%S", seconds (now)=w538, UTC format=FALSE) -> (date/time string=w539:string)
        n121 = Concatenate Strings(w550, "_", w539) -> (w530:string)
        n122 = Build Path(base path=w551, name or relative path=w530) -> (appended path=w552:path)
        n123 = case shown="True" w534 {
          tunnel: w552 -> [w554 w562]
          tunnel: [w555 w557] -> w547
          tunnel: w541 -> [w555 w561]
          tunnel: [w554 w556] -> w529
          frame False {
          }
          frame True {
            n124 = call <vilib>:"Check if File or Folder Exists.vi"("error in (no error)"=w561, "path"=w562) -> ("error out"=w558:errorcluster, "file or folder exists?"=w560:bool, "dup path"=w559:path)  [unwired: 7 in]
            n125 = case shown="False" w560 {
              tunnel: w559 -> [w566 w567]
              tunnel: w558 -> [w565 w568]
              tunnel: [w564 w568] -> w557
              tunnel: [w563 w567] -> w556
              frame False {
                n126 = Create Folder(path (use dialog)=w566, error in=w565) -> (created path=w563:path, error out=w564:errorcluster)  [unwired: 1 in, 1 out]
              }
              frame True {
              }
            }
          }
        }
      }
      frame 7 {
        n127 = Get Queue Status(queue=w587, error in (no error)=w586) -> (queue out=w584:refnum<queue>, error out=w585:errorcluster, # elements in queue=w583:i32)  [unwired: 1 in, 5 out]
        n128 = case shown="True" w582 {
          tunnel: w585 -> [w602 w615]
          tunnel: w584 -> [_ w614]
          tunnel: w583 -> [_ w613]
          tunnel: [w602 w604] -> w581
          tunnel: w580 -> [_ w612]
          tunnel: w579 -> [_ w611]
          tunnel: w578 -> [_ w610]
          tunnel: w576 -> [_ w609]
          tunnel: w575 -> [_ w608]
          tunnel: w574 -> [_ w607]
          tunnel: w573 -> [_ w606]
          tunnel: w570 -> [_ w605]
          tunnel: w569 -> [_ w603]
          frame False {
          }
          frame True {
            n129 = for {
              N: w613 -> [_]
              tunnel: w614 -> [w632]
              tunnel: w615 -> [w631]
              tunnel: w612 -> [w620]
              tunnel: w611 -> [w629]
              tunnel: w610 -> [w628]
              tunnel: w609 -> [w627]
              tunnel: w608 -> [w625]
              tunnel: w607 -> [w624]
              tunnel: w606 -> [w621]
              tunnel: w605 -> [w619]
              tunnel: [w617] -> w604
              tunnel: w603 -> [w616]
              n130 = Dequeue Element(queue=w632, error in (no error)=w631) -> (element=w630:T6, error out=w622:errorcluster)  [unwired: 1 in, 2 out]
              n131 = Unbundle(w630) -> ("ImgDataArray"=w618:u16[][], "Frame No."=w626:i32)  [unwired: 2 out]
              n132 = case shown="True" w627 {
                tunnel: w629 -> [_ w650]
                tunnel: w628 -> [_ w649]
                tunnel: w622 -> [w638 w642]
                tunnel: w626 -> [_ w647]
                tunnel: [w638 w648] -> w623
                tunnel: w618 -> [_ w640]
                tunnel: w621 -> [_ w645]
                tunnel: w620 -> [_ w641]
                tunnel: w619 -> [_ w646]
                tunnel: w616 -> [_ w639]
                frame False {
                }
                frame True {
                  n133 = case shown="7, Default" w641 {
                    tunnel: w640 -> [w653 w664]
                    tunnel: w642 -> [w657 w663]
                    tunnel: [w656 w662] -> w643
                    tunnel: w645 -> [w655 w661]
                    tunnel: [w654 w660] -> w644
                    tunnel: w639 -> [w651 _]
                    frame 0 {
                      n134 = for {
                        workers-P: w651 -> [_]
                        tunnel: [w659] -> w652 mode=indexing
                        tunnel: w653 -> [w658] mode=indexing
                        n135 = To Unsigned Byte Integer(number=w658) -> (unsigned 8bit integer=w659:u8[])
                      }
                      n136 = call "IMAQ ArrayToImage"("error in (no error)"=w657, "Image Pixels (U8)"=w652, "Image"=w655) -> ("error out"=w656:errorcluster, "Image Out"=w654:T4)  [unwired: 7 in]
                    }
                    frame 7, Default {
                      n137 = call "IMAQ ArrayToImage"("Image Pixels (U16)"=w664, "error in (no error)"=w663, "Image"=w661) -> ("error out"=w662:errorcluster, "Image Out"=w660:T4)  [unwired: 7 in]
                    }
                  }
                  n138 = case shown="\"TIFF\", Default" w650 {
                    tunnel: [w675 w680] -> w648
                    tunnel: [w667 w679] -> _
                    tunnel: w644 -> [w669 w678]
                    tunnel: w649 -> [w667 w677]
                    tunnel: w643 -> [w668 w676]
                    tunnel: w647 -> [w666 _]
                    tunnel: w646 -> [w665 _]
                    frame "TIFF", Default {
                      n139 = Format Value(format string="%09d", value (0)=w666) -> (output string=w672:string)  [unwired: 1 in]
                      n140 = Concatenate Strings(w672, ".tiff" ("string")) -> (w671:string)
                      n141 = Build Path(base path=w665, name or relative path=w671) -> (appended path=w670:path)
                      n142 = call-poly "IMAQ Write File 2"("error in (no error)"=w668, "File Path"=w670, "Image"=w669) -> ("error out"=w675:errorcluster)  [unwired: 7 in, 1 out]
                    }
                    frame "AVI" {
                      n143 = call "IMAQ AVI2 Write Frame"("error in (no error)"=w676, "Image"=w678, "AVI Refnum"=w677) -> ("error out"=w680:errorcluster, "AVI Refnum (duplicate)"=w679:T12)  [unwired: 6 in, 1 out]
                    }
                  }
                }
              }
              n144 = case shown="True" w625 {
                tunnel: w624 -> [_ w636]
                tunnel: w623 -> [w633 w637]
                tunnel: w618 -> [_ w635]
                tunnel: [w633 w634] -> w617
                frame False {
                }
                frame True {
                  n145 = Enqueue Element(queue=w636, element=w635, error in (no error)=w637) -> (error out=w634:errorcluster)  [unwired: 1 in, 2 out]
                }
              }
            }
          }
        }
        n146 = Increment(x=w590) -> (x+1=w589:u16)
        n147 = And(x=w582, y=w576) -> (x .and. y?=w588:bool)
        n148 = Read from Binary File(5:0.0, 8:w581, 9:w597, 11:w595) -> (0:w596:errorcluster, 3:w594:refnum<file>)  [unwired: 2 in, 2 out]
        n149 = case shown="True" w588 {
          tunnel: [w681 w685] -> w601
          tunnel: w596 -> [w681 w684]
          tunnel: w579 -> [_ w683]
          tunnel: w578 -> [_ w682]
          frame False {
          }
          frame True {
            n150 = case shown="\"AVI\"" w683 {
              tunnel: [w686 w689] -> w685
              tunnel: w684 -> [w686 w688]
              tunnel: w682 -> [_ w687]
              frame "TIFF", Default {
              }
              frame "AVI" {
                n151 = call "IMAQ AVI2 Close"("error in (no error)"=w688, "AVI Refnum"=w687) -> ("error out"=w689:errorcluster)  [unwired: 9 in]
              }
            }
          }
        }
      }
    }
    "Frame Rate" <- w128
    n152 = Get File Position(4:w120, 7:w121) -> (0:w118:errorcluster, 2:w101:i64, 3:w119:refnum<file>)
    n153 = Divide(x=w101, y=w100) -> (x/y=→"Progress":dbl)
    n154 = Greater?(x=w100, y=w101) -> (0:w117:bool)
    n155 = Not(x=w117) -> (.not. x?=w92:bool)
    n156 = case shown="True" w117 {
      tunnel: w132 -> [_ w146]
      tunnel: [u8 0 w145] -> w130
      tunnel: [w139 w144] -> w80
      tunnel: w119 -> [w138 w143]
      tunnel: w118 -> [w139 w142]
      tunnel: [w138 w141] -> w98
      frame False {
      }
      frame True {
        n157 = Read from Binary File(5:u8 0, 8:w142, 9:w146, 11:w143) -> (0:w144:errorcluster, 2:w145:u8, 3:w141:refnum<file>)  [unwired: 2 in, 1 out]
      }
    }
    n158 = Or(x=w92, y="Stop") -> (x .or. y?=w78:bool)
    n159 = Unbundle By Name(w80) -> ("status"=w79:bool)
    n160 = Or(x=w79, y=w78) -> (x .or. y?=w77:bool)
    "Sequence No." <- w127
    "Frame No." <- w85
  }
  n161 = Close File(refnum=w46, error in=w47) -> (error out=w42:errorcluster)  [unwired: 1 out]
  n162 = Unbundle By Name("Input Parameters") -> ("Timeout for Queue(ms)"=w31:u32)
  n163 = call "Imaq Dispose"("All Images? (No)"=TRUE, "error in (no error)"=w42) -> ("error out"=w41:errorcluster)  [unwired: 4 in]
  n164 = while {
    tunnel: w35 -> [w700]
    tunnel: w41 -> [w699]
    tunnel: [w698] -> w39
    tunnel: [w697] -> w40
    shift-right: [w694] -> _
    shift-left: 0 ("# elements in queue") -> [w695]
    tunnel: w31 -> [w690]
    stop <- w691 stop-if-true
    n165 = Get Queue Status(queue=w700, error in (no error)=w699) -> (queue out=w697:refnum<queue>, error out=w698:errorcluster, # elements in queue=w694:i32)  [unwired: 1 in, 5 out]
    n166 = Equal?(x=w694, y=0) -> (x = y?=w692:bool)
    n167 = Equal?(x=w694, y=w695) -> (x = y?=w693:bool)
    n168 = Or(x=w693, y=w692) -> (x .or. y?=w691:bool)
    n169 = Wait (ms)(milliseconds to wait=w690) -> ()  [unwired: 1 out]
  }
  n170 = Flush Queue(queue=w40, error in (no error)=w39) -> (queue out=w37:refnum<queue>, error out=w38:errorcluster)  [unwired: 1 out]
  n171 = Release Queue(queue=w37, error in (no error)=w38) -> (error out=w8:errorcluster)  [unwired: 1 in, 2 out]
  n172 = Release Queue(queue=w9, error in (no error)=w8) -> (error out=→"error out":errorcluster)  [unwired: 1 in, 2 out]
